vi "AttackerBurro.vi"(9 "balls":T1[](array[typedef]), 10 "Field Size in":T3, 11 "Robot in":T2) -> (3 "Robot out":T2)   [LabVIEW 2016]
uses:
  Core/Field Size.ctl
  Core/AI Robot.ctl
  Core/AI Ball.ctl
  <vilib>/Analysis/_algsub.llb/Real Vector Norm.vi
  <vilib>/Analysis/NI_AALPro.lvlib
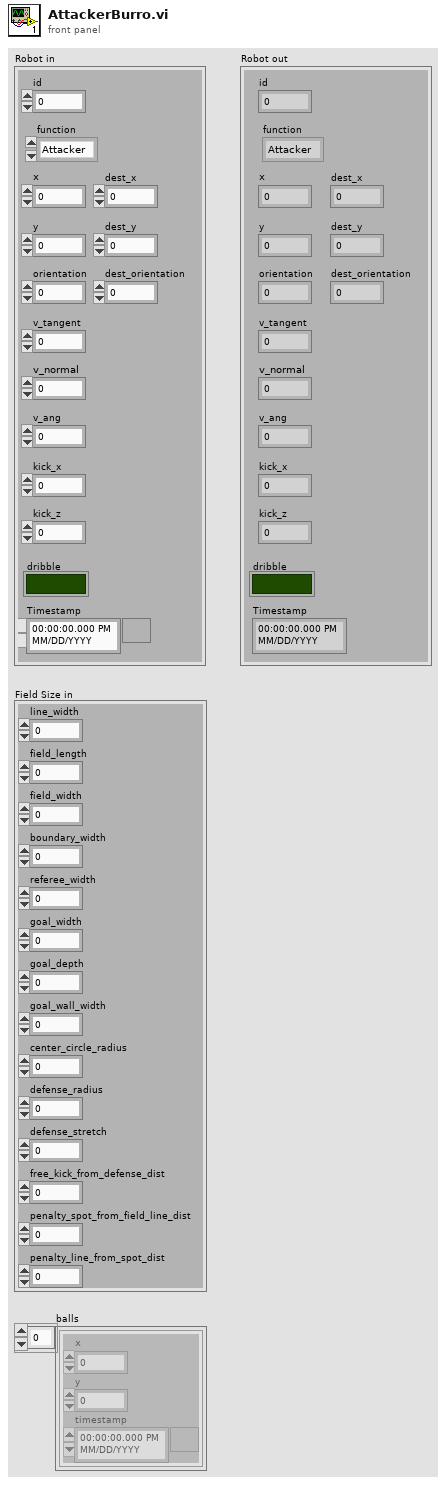
[diagram p1: front panel]
types:
  T1 = typedef "AI Ball.ctl" = cluster{"x":dbl, "y":dbl, "timestamp":timestamp}
  T2 = typedef "AI Robot.ctl" = cluster{"id":u32, "function":enum16{"Attacker", "Goalie", "Defender"}, "x":dbl, "y":dbl, "orientation":dbl, "v_tangent":dbl, "v_normal":dbl, "v_ang":dbl, "kick_x":dbl, "kick_z":dbl, "dribble":bool, "Timestamp":timestamp, "dest_x":dbl, "dest_y":dbl, "dest_orientation":dbl}
  T3 = typedef "Field Size.ctl" = cluster{"line_width":u32, "field_length":u32, "field_width":u32, "boundary_width":u32, "referee_width":u32, "goal_width":u32, "goal_depth":u32, "goal_wall_width":u32, "center_circle_radius":u32, "defense_radius":u32, "defense_stretch":u32, "free_kick_from_defense_dist":u32, "penalty_spot_from_field_line_dist":u32, "penalty_line_from_spot_dist":u32}
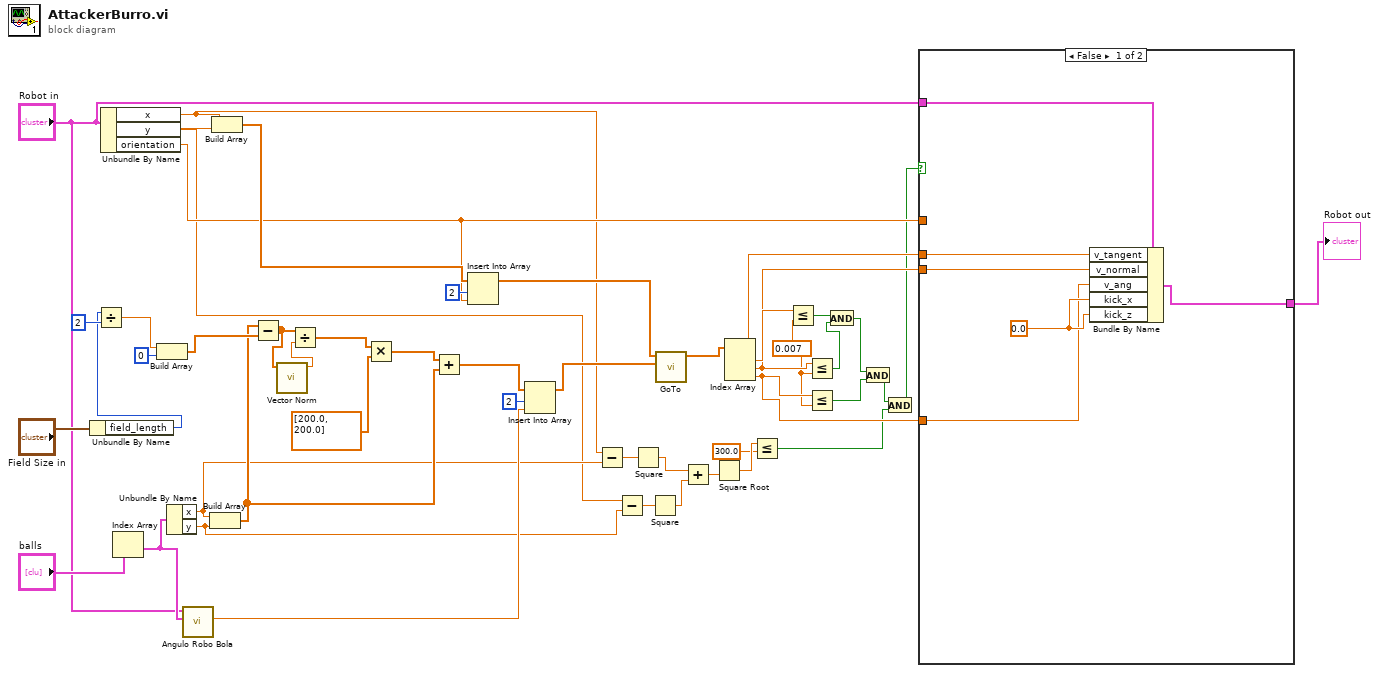
[diagram p0: block diagram]
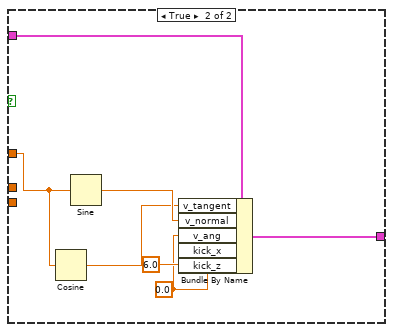
[diagram p2: hidden frame]
diagram:
  w16 = 0.007
  n1 = Unbundle By Name("Field Size in") -> ("field_length"=w45:u32)
  n2 = Divide(x=w45, y=u32 2) -> (x/y=w47:dbl)
  n3 = Unbundle By Name("Robot in") -> ("x"=w14:dbl, "y"=w10:dbl, "orientation"=w23:dbl)
  n4 = Index Array(array="balls") -> (element=w32:T1)  [unwired: 1 in]
  n5 = Build Array(w47, u32 0 ("element")) -> (w44:dbl[])
  n6 = Unbundle By Name(w32) -> ("x"=w13:dbl, "y"=w9:dbl)
  n7 = call "Angulo Robo Bola.vi"("Ball"=w32, "Robot"="Robot in") -> ("Angulo"=w39:dbl)  [unwired: 9 in]
  n8 = Build Array(w13, w9) -> (w42:dbl[])
  n9 = Build Array(w14, w10) -> (w35:dbl[])
  n10 = Subtract(x=w42, y=w44) -> (x-y=w27:dbl[])
  n11 = call-poly <vilib>:"Vector Norm.vi"("Input Vector"=w27) -> ("norm"=w28:dbl)  [unwired: 9 in, 1 out]
  n12 = Divide(x=w27, y=w28) -> (x/y=w29:dbl[])
  n13 = Multiply(x=w29, y=dbl[] [200.0, 200.0]) -> (x*y=w31:dbl[])
  n14 = Add(x=w31, y=w42) -> (x+y=w38:dbl[])
  n15 = Insert Into Array(array=w35, index=2, new element=w23) -> (w36:dbl[])
  n16 = Insert Into Array(array=w38, index=2, new element=w39) -> (w40:dbl[])
  n17 = Subtract(x=w14, y=w13) -> (x-y=w12:dbl)
  n18 = Subtract(x=w10, y=w9) -> (x-y=w11:dbl)
  n19 = Square(x=w12) -> (x^2=w8:dbl)
  n20 = Square(x=w11) -> (x^2=w7:dbl)
  n21 = call "GoTo.vi"("Target"=w40, "Position"=w36) -> ("Output\nVelocity"=w33:dbl[])  [unwired: 9 in]
  n22 = Add(x=w8, y=w7) -> (x+y=w6:dbl)
  n23 = Square Root(x=w6) -> (sqrt(x)=w5:dbl)
  n24 = Index Array(array=w33) -> (element #1=w19:dbl, element #2=w18:dbl, element #3=w17:dbl)  [unwired: 3 in]
  n25 = Less Or Equal?(x=w5, y=300.0) -> (x <= y?=w2:bool)
  n26 = Less Or Equal?(x=w19, y=w16) -> (x <= y?=w21:bool)
  n27 = Less Or Equal?(x=w18, y=w16) -> (x <= y?=w20:bool)
  n28 = Less Or Equal?(x=w17, y=w16) -> (x <= y?=w15:bool)
  n29 = And(x=w21, y=w20) -> (x .and. y?=w25:bool)
  n30 = And(x=w25, y=w15) -> (x .and. y?=w4:bool)
  n31 = And(x=w4, y=w2) -> (x .and. y?=w1:bool)
  n32 = case shown="False" w1 {
    tunnel: "Robot in" -> [w48 w60]
    tunnel: w23 -> [_ w57]
    tunnel: [w49 w54] -> w22
    tunnel: w17 -> [w52 _]
    tunnel: w18 -> [w51 _]
    tunnel: w19 -> [w50 _]
    frame False {
      w53 = 0.0 ("kick_x")
      n33 = Bundle By Name(cluster=w48, "v_tangent"=w50, "v_normal"=w51, "v_ang"=w52, "kick_x"=w53, "kick_z"=w53) -> (w49:T2)
    }
    frame True {
      w58 = 0.0 ("kick_z")
      n34 = Cosine(x=w57) -> (cos(x)=w55:dbl)
      n35 = Sine(x=w57) -> (sin(x)=w56:dbl)
      n36 = Bundle By Name(cluster=w60, "v_tangent"=w55, "v_normal"=w56, "v_ang"=w58, "kick_x"=6.0, "kick_z"=w58) -> (w54:T2)
    }
  }
  "Robot out" <- w22
